vi "LIA 4HF Decimators.vi"(5 "clock x 2":refnum<k21>, 7 "reset":bool, 9 "input valid":bool, 11 "data in":T1) -> (1 "output valid":bool, 3 "data out":T1)   [LabVIEW 2018]
uses:
  <instrlib>/_niInstr/DSP/v1/Shared/Public/IQ Data.ctl
  <instrlib>/_niInstr/DSP/v1/FPGA/Public/Sub VIs/HB Decimator/Halfband Decimator - IQ - 1 SPC - 2x OC.vi
  <instrlib>/_niInstr/DSP/v1/FPGA/niInstr DSP v1 FPGA.lvlib
  <instrlib>/_niInstr/DSP/v1/Shared/niInstr DSP v1 Shared.lvlib
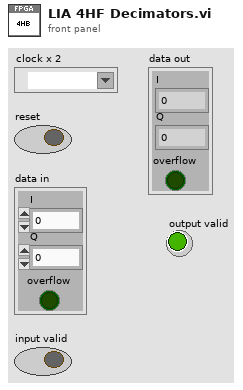
[diagram p1: front panel]
types:
  T1 = typedef "niInstr DSP v1 Shared.lvlib/IQ Data.ctl" = cluster{"I":fxp<+/-,18,1>, "Q":fxp<+/-,18,1>, "overflow":bool}
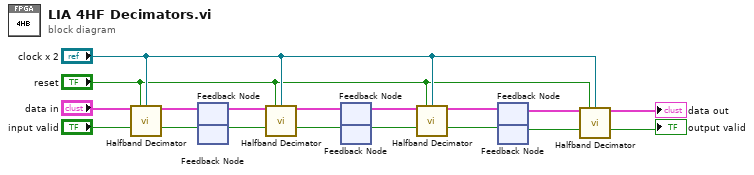
[diagram p0: block diagram]
diagram:
  n1 = call-poly <instrlib>:"Halfband Decimator.vi"("data in"="data in", "reset"="reset", "clock x 2"="clock x 2", "input valid"="input valid") -> ("data out"=w16:T1, "output valid"=w15:bool)  [unwired: 8 in, 2 out]
  n2 = feedback-in #1(w16) -> ()
  n3 = feedback #1() -> (w6:T1)  [unwired: 1 in]
  n4 = feedback-in #2(w15) -> ()
  n5 = feedback #2() -> (w5:bool)  [unwired: 1 in]
  n6 = call-poly <instrlib>:"Halfband Decimator.vi"("data in"=w6, "reset"="reset", "clock x 2"="clock x 2", "input valid"=w5) -> ("data out"=w13:T1, "output valid"=w9:bool)  [unwired: 8 in, 2 out]
  n7 = feedback-in #3(w13) -> ()
  n8 = feedback #3() -> (w4:T1)  [unwired: 1 in]
  n9 = feedback-in #4(w9) -> ()
  n10 = feedback #4() -> (w3:bool)  [unwired: 1 in]
  n11 = call-poly <instrlib>:"Halfband Decimator.vi"("data in"=w4, "reset"="reset", "clock x 2"="clock x 2", "input valid"=w3) -> ("data out"=w11:T1, "output valid"=w8:bool)  [unwired: 8 in, 2 out]
  n12 = feedback-in #5(w11) -> ()
  n13 = feedback #5() -> (w2:T1)  [unwired: 1 in]
  n14 = feedback-in #6(w8) -> ()
  n15 = feedback #6() -> (w1:bool)  [unwired: 1 in]
  n16 = call-poly <instrlib>:"Halfband Decimator.vi"("data in"=w2, "reset"="reset", "clock x 2"="clock x 2", "input valid"=w1) -> ("data out"=→"data out":T1, "output valid"=→"output valid":bool)  [unwired: 8 in, 2 out]
